vi "Apply Force To Position.vi"(8 "Error In":errorcluster, 11 "Display Element In":refnum<class "Display Element.lvclass">) -> (0 "Error Out":errorcluster, 3 "Display Element Out":refnum<class "Display Element.lvclass">)   [LabVIEW 2019, in "Display Element.lvclass"]
uses:
  Display Element.lvclass
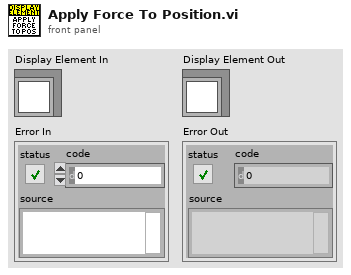
[diagram p1: front panel]
types:
  T1 = typedef "Display Element.lvclass/Vector.ctl" = cluster{"X":i32, "Y":i32}
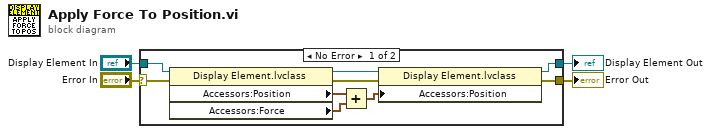
[diagram p0: block diagram]
diagram:
  n1 = case shown="No Error" "Error In" {
    selector: "Error In" -> [w12 w14]
    tunnel: "Display Element In" -> [w10 w15]
    tunnel: [w11 w14] -> w2
    tunnel: [w5 w15] -> w1
    frame No Error {
      n2 = property class="Display Element.lvclass"(reference=w10, error in=w12) -> (reference out=w9:refnum<class "Display Element.lvclass">, error out=w13:errorcluster, "Accessors:Position"=w8:T1, "Accessors:Force"=w7:T1)
      n3 = Add(x=w8, y=w7) -> (x+y=w6:T1)
      n4 = property class="Display Element.lvclass"(reference=w9, error in=w13, "Accessors:Position"=w6) -> (reference out=w5:refnum<class "Display Element.lvclass">, error out=w11:errorcluster)
    }
    frame Error {
    }
  }
  "Display Element Out" <- w1
  "Error Out" <- w2
